vi "StopRumble.vi"(11 "Controller Name":string="My Joystick RefNum") -> ()   [LabVIEW 2020]
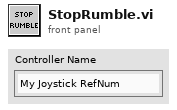
[diagram p1: front panel]
types:
  T1 = typedef "WPI_JoystickDevRef.ctl" = cluster{"Device":T2}
  T2 = typedef "WPI_JoystickDeviceEnum.ctl" = enum16{"USB 0", "USB 1", "USB 2", "USB 3", "USB 4", "USB 5"}
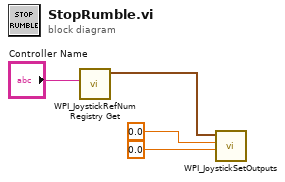
[diagram p0: block diagram]
diagram:
  n1 = call <vilib>:"WPI_JoystickRefNum Registry Get.vi"("refnum name"="Controller Name") -> ("JoystickDevRef"=w3:T1)  [unwired: 1 in, 9 out]
  n2 = call <vilib>:"WPI_JoystickSetOutputs.vi"("Right Rumble"=sgl 0.0, "Left Rumble"=sgl 0.0, "JoystickDevRef"=w3) -> ()  [unwired: 7 in, 2 out]
